vi "Read Roles.vi"(8 "error in (no error)":errorcluster, 11 "Play_v2 in":refnum<class "Play_v2.lvclass">) -> (0 "error out":errorcluster, 2 "Roles":refnum<class "Role_v2.lvclass">[](array[class]), 3 "Play_v2 out":refnum<class "Play_v2.lvclass">)   [LabVIEW 2023, in "Play_v2.lvclass"]
uses:
  Play_v2.lvclass
  NewRoles/Role_v2_class/Role_v2.lvclass
  Play_v2.lvclass/Play_v2.ctl
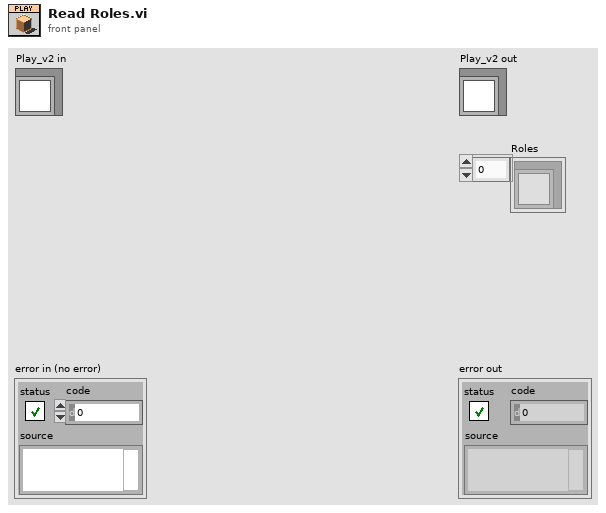
[diagram p1: front panel]
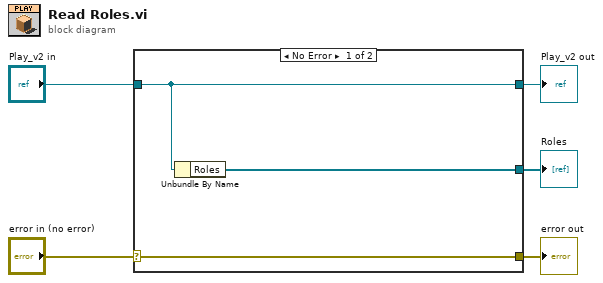
[diagram p0: block diagram]
diagram:
  n1 = case shown="No Error" "error in (no error)" {
    selector: "error in (no error)" -> [w8 w9]
    tunnel: [w8 w9] -> w4
    tunnel: [w7 w10] -> w2
    tunnel: "Play_v2 in" -> [w7 w10]
    tunnel: [w6 _] -> w1
    frame No Error {
      n2 = Unbundle By Name(w7) -> ("Roles"=w6:refnum<class "Role_v2.lvclass">[])
    }
    frame Error {
    }
  }
  "error out" <- w4
  "Play_v2 out" <- w2
  "Roles" <- w1
